vi "set_led_enable.vi"(8 "error in":errorcluster, 9 "I2C interface":T1, 11 "LED enables":bool[](array[boolean])=[TRUE, TRUE, TRUE, TRUE, TRUE, TRUE]) -> (0 "error out":errorcluster)   [LabVIEW 2014]
uses:
  i2c_interface.ctl
  fpga_reference.ctl
  <vilib>/Utility/error.llb/Error Cluster From Error Code.vi
  <vilib>/rvi/errors/niLvFpgaAdjustHostInterfaceError.vi
  <vilib>/rvi/interface/nirviReadWriteControl/nirviReadWriteControl.xnode
  FPGA Bitfiles/i2cmuxdemux.lvbitx
  NiFpgaLv.dll
panel:
  # "Set output enables for ASAP LEDs.  Useful for switching off some lights for testing."
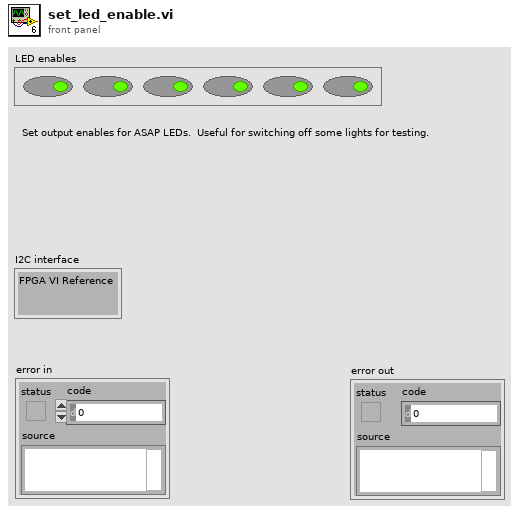
[diagram p1: front panel]
types:
  T1 = typedef "i2c_interface.ctl" = cluster{"FPGA VI Reference":T2}
  T2 = typedef "fpga_reference.ctl" = refnum<k20>
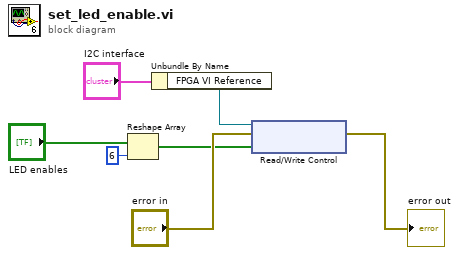
[diagram p0: block diagram]
diagram:
  n1 = Reshape Array("LED enables", 6 ("dimension size")) -> (w1:bool[])
  n2 = Unbundle By Name("I2C interface") -> ("FPGA VI Reference"=w4:T2)
  n3 = xnode "Read/Write Control"("FPGA VI Reference In"=w4, "error in"="error in", "Output enable"=w1) -> ("error out"=→"error out":errorcluster)  [unwired: 1 out]
